vi "Set Laser Power Reply.vi"(8 "error in (no error)":errorcluster, 11 "Application in":refnum<class "Application.lvclass">) -> (0 "error out":errorcluster, 3 "Application out":refnum<class "Application.lvclass">)   [LabVIEW 2023, in "Application.lvlib" / "Application.lvclass"]
uses:
  Application.lvclass
  Application.lvclass/Application.ctl
  Mode.ctl
  Application.lvlib
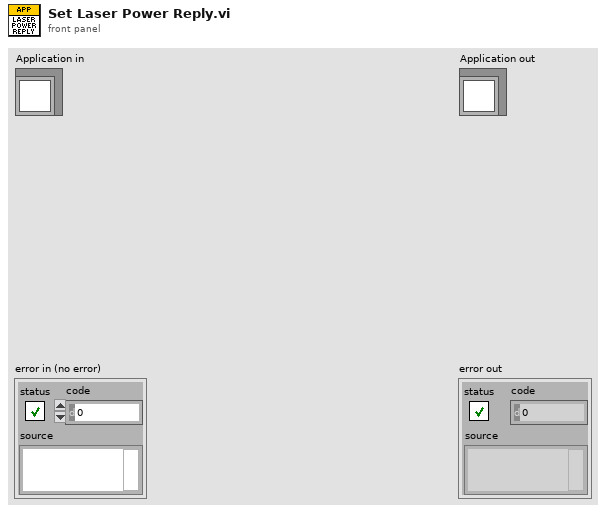
[diagram p1: front panel]
types:
  T1 = typedef "Application.lvlib/Mode.ctl" = enum16{"Idle", "Cancel", "Live", "Stream", "Autofocus", "Z-Stack", "Montage", "Saving", "Stage Scan", "Laser Adjust"}
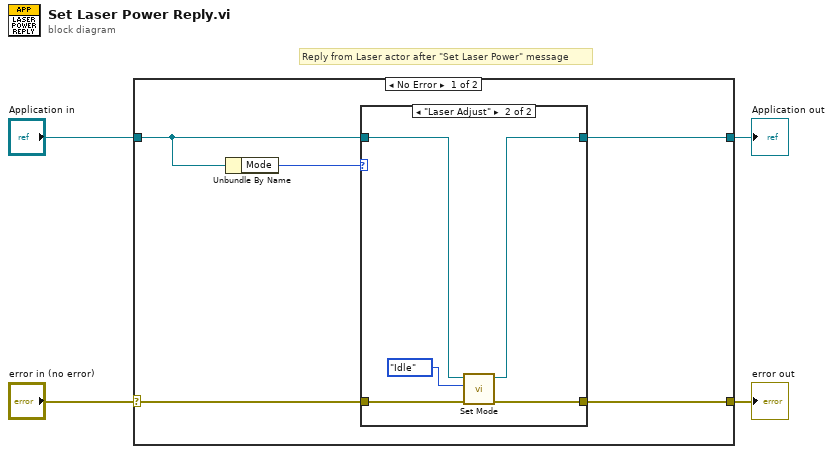
[diagram p0: block diagram]
diagram:
  # "Reply from Laser actor after \"Set Laser Power\" message"
  n1 = case shown="No Error" "error in (no error)" {
    selector: "error in (no error)" -> [w9 w18]
    tunnel: [w8 w18] -> w3
    tunnel: [w7 w17] -> w1
    tunnel: "Application in" -> [w6 w17]
    frame No Error {
      n2 = Unbundle By Name(w6) -> ("Mode"=w5:T1)
      n3 = case shown="\"Laser Adjust\"" w5 {
        tunnel: w9 -> [w11 w14]
        tunnel: [w11 w13] -> w8
        tunnel: w6 -> [w10 w16]
        tunnel: [w10 w15] -> w7
        frame Default {
        }
        frame "Laser Adjust" {
          n4 = call-dynamic "Set Mode.vi"("error in (no error)"=w14, "New Mode"=Mode."Idle", "Application in"=w16) -> ("error out"=w13:errorcluster, "Application out"=w15:refnum<class "Application.lvclass">)  [unwired: 7 in]
        }
      }
    }
    frame Error {
    }
  }
  "error out" <- w3
  "Application out" <- w1
